vi "Scan_Set_up_OPO.vi"() -> (0 "Array":string[][](array[string]), 1 "Scan List":i32(listbox), 2 "ScanPoints":dbl[](array[numeric]), 5 "Cancelled?":bool)   [LabVIEW 2019]
panel:
  in  "Number of Points":dbl
  in  "CmdCancel":bool
  in  "CmdOK":bool
  in  "Log Scale?":bool
  in  "Scan End / nm":dbl
  in  "Scan Start / nm":dbl
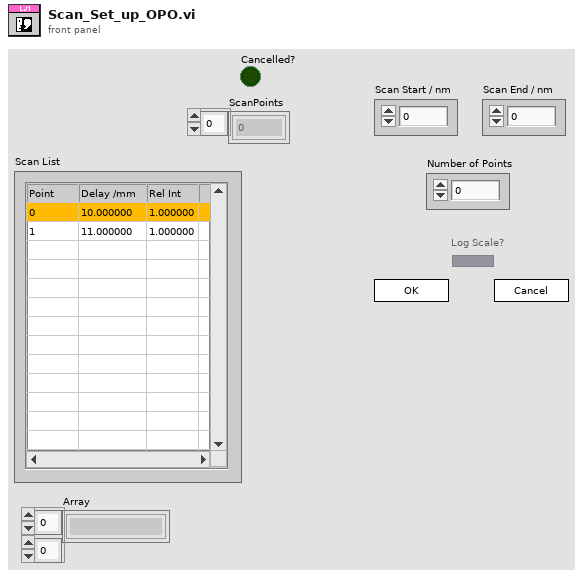
[diagram p1: front panel]
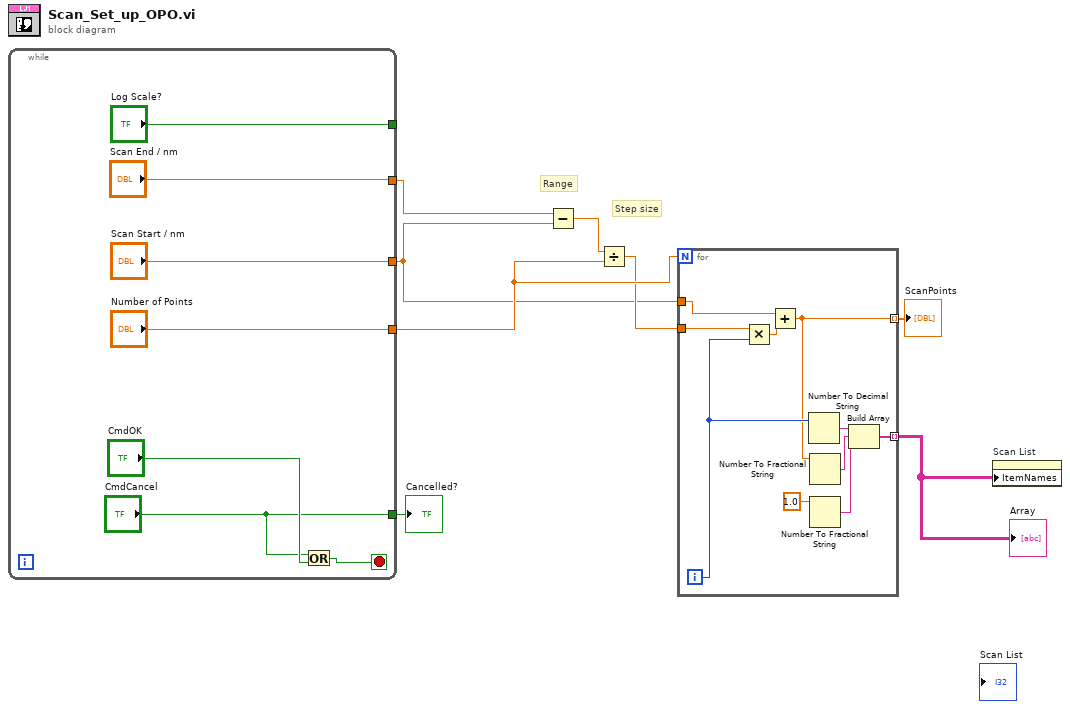
[diagram p0: block diagram]
diagram:
  # "Step size"
  # "Range"
  n1 = while {
    tunnel: ["CmdCancel"] -> w8
    tunnel: ["Scan Start / nm"] -> w2
    tunnel: ["Scan End / nm"] -> w6
    tunnel: ["Log Scale?"] -> _
    tunnel: ["Number of Points"] -> w4
    stop <- w14 stop-if-true
    n2 = Or(x="CmdCancel", y="CmdOK") -> (x .or. y?=w14:bool)
  }
  "Cancelled?" <- w8
  n3 = Subtract(x=w6, y=w2) -> (x-y=w7:dbl)
  n4 = Divide(x=w7, y=w4) -> (x/y=w3:dbl)
  n5 = for {
    N: w4 -> [_]
    tunnel: w3 -> [w24]
    tunnel: w2 -> [w25]
    tunnel: [w19] -> w5 mode=indexing
    tunnel: [w20] -> w1 mode=indexing
    i -> [w22]
    n6 = Multiply(x=w24, y=w22) -> (x*y=w23:dbl)
    n7 = Add(x=w25, y=w23) -> (x+y=w19:dbl)
    n8 = Number To Decimal String(number=w22) -> (decimal integer string=w21:string)  [unwired: 1 in]
    n9 = Number To Fractional String(number=w19) -> (F-format string=w18:string)  [unwired: 3 in]
    n10 = Number To Fractional String(number=1.0) -> (F-format string=w16:string)  [unwired: 3 in]
    n11 = Build Array(w21, w18, w16) -> (w20:string[])
  }
  "ScanPoints" <- w5
  "Array" <- w1
  n12 = property on="Scan List" class="MCListbox (strict)"("ItemNames"=w1) -> ()  [unwired: 2 in, 2 out]
